vi "TA Main - Copy.vi"() -> ()   [LabVIEW 2019]
doc: "This example demonstrates how to acquire a continuous amount of data (Waveform) using the DAQ device's internal clock. It also shows how to synchronize two devices for different device families (E Series, S Series, M Series, X Series, DSA, and SC Express), to simultaneously acquire the data.\n\nFor instructions on how to connect your signals to the DAQ device, refer to your device documentation."
uses:
  Program Files/National Instruments/LabVIEW 2019/examples/Instrument IO/Serial/support/Serial - Settings.ctl
  <vilib>/Utility/error.llb/DialogType.ctl
  <vilib>/DAQmx/read.llb/DAQmx Read (Analog 1D Wfm NChan NSamp).vi
  <vilib>/Instr/_visa.llb/VISA Configure Serial Port (Instr).vi
  <vilib>/DAQmx/configure/timing.llb/DAQmx Timing (Sample Clock).vi
  <vilib>/DAQmx/configure/trigger.llb/DAQmx Start Trigger (Digital Edge).vi
  <vilib>/DAQmx/miscellaneous.llb/DAQmx Fill In Error Info.vi
panel:
  in  "Pass Logger":T1(tab)
  out "CO2 chart":waveform(dbl)[](graph)=[{"t0"=timestamp(3665042798.734879 s since 1904-01-01), "dt"=0.0, "Y"=[151.0], "attributes"=variant("NI_ChannelName"=variant(string "SCD30 CO2"), "NI_UnitDescription"=variant(string "ppm"))}, {"t0"=timestamp(3665042798.734879 s since 1904-01-01), "dt"=0.0, "Y"=[28.44], "attributes"=variant("NI_ChannelName"=variant(string "SCD30 Temp"), "NI_UnitDescription"=variant(string "C"))}, {"t0"=timestamp(3665042798.734879 s since 1904-01-01), "dt"=0.0, "Y"=[0.0], "attributes"=variant("NI_ChannelName"=variant(string "SCD30 Humidity"), "NI_UnitDescription"=variant(string "%"))}]
  in  "Stop":bool
  in  "Enable logging":bool caption="Enable"
  in  "File config":T2={"Filepath"=path "C:/Users/Administrator/Desktop/DAQ TA/Test data", "Test ID"="CO2_pulse_test_50sscm_1v5", "PC"="69DTQV2"}
  out "Lockin chart":waveform(dbl)[](graph)=[{"t0"=timestamp(3665042794.5437593 s since 1904-01-01), "dt"=4.999, "Y"=[-0.0029492353085881725], "attributes"=variant("NI_ChannelName"=variant(string "Phase - Mic Diff"), "NI_UnitDescription"=variant(string "Rad"))}, {"t0"=timestamp(3665042794.5437593 s since 1904-01-01), "dt"=4.999, "Y"=[2.2024304960006402], "attributes"=variant("NI_ChannelName"=variant(string "Amplitude - Mic Diff"), "NI_UnitDescription"=variant(string "Volts"))}]
  out "Lockin output 1":T3={"X"=1.1012104588247866, "Y"=-0.0032477381836216656, "R"=1.1012152480003201, "θ"=-0.0029492353085881725, "Amp"=2.2024304960006402, "dt"=4.999, "Active channel"="Mic Diff", "Ref channel"="Heater Voltage"} {"X" format="%#_3g"; "Y" format="%#_3g"; "R" format="%#_3g"}
  in  "Sampling config":cluster{"Fs":dbl, "#s":dbl}={"Fs"=1000.0, "#s"=5000.0} {"Fs" format="%.2p"}
  out "Readings":T4={"SCD30 CO2"=220.0, "SCD30 Temp (C)"=28.44, "SCD30 RH (%)"=0.0}
  out "Enable logging":bool
  in  "CO2 offset":dbl=69.0
  in  "Config 1":cluster{"Ref Index":i32, "Active Index":i32}={"Ref Index"=2, "Active Index"=5}
  out "Lockin output 5":T3={"X"=7.331709643282483, "Y"=0.49731099109465005, "R"=7.348556628023282, "θ"=0.06772641255423814, "Amp"=14.697113256046563, "dt"=4.999, "Active channel"="Heater Current", "Ref channel"="Heater Voltage"} {"X" format="%#_3g"; "Y" format="%#_3g"; "R" format="%#_3g"}
  out "Lockin output 6":T3={"X"=10.405708679082442, "Y"=0.4366095430141891, "R"=10.414864425761035, "θ"=0.04193405807955491, "Amp"=20.82972885152207, "dt"=4.999, "Active channel"="Heater Power", "Ref channel"="Heater Voltage"} {"X" format="%#_3g"; "Y" format="%#_3g"; "R" format="%#_3g"}
  out "Lockin output 4":T3={"X"=0.3532460188223979, "Y"=-0.0002886373096321914, "R"=0.35324613674514604, "θ"=-0.0008170997831991877, "Amp"=0.7064922734902921, "dt"=4.999, "Active channel"="Heater Voltage", "Ref channel"="Heater Voltage"} {"X" format="%#_3g"; "Y" format="%#_3g"; "R" format="%#_3g"}
  out "Lockin output 3":T3={"X"=1.1011542239382506, "Y"=-0.0034004178869849783, "R"=1.101159474253778, "θ"=-0.003088038899800522, "Amp"=2.202318948507556, "dt"=4.999, "Active channel"="Mic Active", "Ref channel"="Heater Voltage"} {"X" format="%#_3g"; "Y" format="%#_3g"; "R" format="%#_3g"}
  out "Lockin output 2":T3={"X"=-5.629936956115632e-05, "Y"=-0.00017491984854744577, "R"=0.00018375682961143246, "θ"=-1.8821838626707943, "Amp"=0.0003675136592228649, "dt"=4.999, "Active channel"="Mic Ref", "Ref channel"="Heater Voltage"} {"X" format="%#_3g"; "Y" format="%#_3g"; "R" format="%#_3g"}
  in  "Config 5":cluster{"Ref Index":i32, "Active Index":i32}={"Ref Index"=2, "Active Index"=6}
  in  "Config 4":cluster{"Ref Index":i32, "Active Index":i32}={"Ref Index"=2, "Active Index"=2}
  in  "Config 3":cluster{"Ref Index":i32, "Active Index":i32}={"Ref Index"=2, "Active Index"=1}
  in  "Config 2":cluster{"Ref Index":i32, "Active Index":i32}={"Ref Index"=2, "Active Index"=0}
  in  "Config 6":cluster{"Ref Index":i32, "Active Index":i32}={"Ref Index"=2, "Active Index"=8}
  out "Lockin output 1":T3={"X"=1.1012104588247866, "Y"=-0.0032477381836216656, "R"=1.1012152480003201, "θ"=-0.0029492353085881725, "Amp"=2.2024304960006402, "dt"=4.999, "Active channel"="Mic Diff", "Ref channel"="Heater Voltage"} {"X" format="%#_3g"; "Y" format="%#_3g"; "R" format="%#_3g"}
  in  "Config 7":cluster{"Ref Index":i32, "Active Index":i32}={"Ref Index"=2, "Active Index"=9}
  out "Lockin output 7":T3={"X"=5.973852436849716, "Y"=-22.75873151918968, "R"=23.529699813210815, "θ"=-1.3141009280278624, "Amp"=47.05939962642163, "dt"=4.999, "Active channel"="Heater Temp", "Ref channel"="Heater Voltage"} {"X" format="%#_3g"; "Y" format="%#_3g"; "R" format="%#_3g"}
  in  "Config 8":cluster{"Ref Index":i32, "Active Index":i32}={"Ref Index"=2, "Active Index"=7}
  out "Lockin output 8":T3={"X"=0.4029293718854757, "Y"=-1.4812546309068166, "R"=1.535078942696731, "θ"=-1.3052036543950893, "Amp"=3.070157885393462, "dt"=4.999, "Active channel"="Heater Resistance", "Ref channel"="Heater Voltage"} {"X" format="%#_3g"; "Y" format="%#_3g"; "R" format="%#_3g"}
  out "Lockin output 9":T3={"X"=-0.008023964066543083, "Y"=0.030564692860772787, "R"=0.03160038684912812, "θ"=1.8275270682644151, "Amp"=0.06320077369825625, "dt"=4.999, "Active channel"="Diode Voltage", "Ref channel"="Heater Voltage"} {"X" format="%#_3g"; "Y" format="%#_3g"; "R" format="%#_3g"}
  in  "Config 9":cluster{"Ref Index":i32, "Active Index":i32}={"Ref Index"=2, "Active Index"=4}
  in  "VISA resource name 2":refnum<visa-resource-name>="COM6"
  in  "Serial Settings":T5={"baud rate"=9600, "data bits"=8, "parity"=enum."None", "stop bits"=10, "flow control"=0} {"flow control" items=["None"=0, "XON/XOFF"=1, "RTS/CTS"=2, "DTR/DSR"=4]; "stop bits" items=["1.0"=10, "1.5"=15, "2.0"=20]; "data bits" min=5 max=8 step=1; "baud rate" items=["75"=75, "110"=110, "134"=134, "150"=150, "300"=300, "600"=600, "1200"=1200, "1800"=1800, "2400"=2400, "4800"=4800, "7200"=7200, "9600"=9600, "14400"=14400, "19200"=19200, "28800"=28800, "38400"=38400, "56000"=56000, "57600"=57600, "115200"=115200, "128000"=128000, "230400"=230400]}
  out "Waveform":waveform(dbl)(graph)={"t0"=timestamp(3665042794.5437374 s since 1904-01-01), "dt"=0.001, "Y"=array[5000 elements], "attributes"=variant("NI_ChannelName"=variant(string "Mic Diff"), "NI_UnitDescription"=variant(string "Volts"))}
  out "Channel names":T6={"Ref channel"="Mic Ref", "Active channel"="Mic Active"}
  in  "Config":T7={"Ref Index"=0, "Active Index"=1, "Gain"=1.0, "Channel name"="Mic Diff", "Enable"=TRUE, "Offset"=0.0035}
  in  "Filter config":T8={"Lower Cut-Off"=49.0, "Upper Cut-Off"=51.0}
  out "Noise estimate (mVrms)":dbl=53.14761345113184 format="%0.2f"
  out "Channel name":string="Diode Voltage"
  in  "Config":T9={"Channel Index"=4, "Diode TC (mV)"=-1.343, "Channel name"="Heater Temp", "Ref voltage"=0.8536, "Ref temp"=25.0} {"Ref temp" format="%.3f"; "Ref voltage" format="%.3f"; "Diode TC (mV)" format="%.3f"}
  out "AO Waveform Graph":waveform(dbl)(graph)={"t0"=timestamp(0 s since 1904-01-01), "dt"=0.001, "Y"=array[5000 elements]}
  in  "Channel config":T10={"Frequency"=47.0, "Voltage"=1.5, "Signal type"=enum."Sine Wave", "Square wave duty cycle (%)"=50.0, "physical channels"="Dev1/ao0", "name to assign"="Heater Voltage", "Phase"=-90.0} {"Square wave duty cycle (%)" format="%0.2f"}
  in  "Config":T11={"Voltage channel index"=2, "Shunt channel index"=3, "Shunt resistance"=10}
  out "Channel names":T12={"Voltage channel name"="Heater Voltage", "Shunt channel name"="Heater Shunt"}
  out "Diode Waveform":waveform(dbl)[](graph)=[{"t0"=timestamp(3665042794.5437374 s since 1904-01-01), "dt"=0.001, "Y"=array[5000 elements], "attributes"=variant("NI_ChannelName"=variant(string "Mic Ref"), "NI_UnitDescription"=variant(string "Volts"))}, {"t0"=timestamp(3665042794.5437484 s since 1904-01-01), "dt"=0.001, "Y"=array[5000 elements], "attributes"=variant("NI_ChannelName"=variant(string "Mic Active"), "NI_UnitDescription"=variant(string "Volts"))}, {"t0"=timestamp(3665042794.5437593 s since 1904-01-01), "dt"=0.001, "Y"=array[5000 elements], "attributes"=variant("NI_ChannelName"=variant(string "Heater Voltage"), "NI_UnitDescription"=variant(string "Volts"))}, {"t0"=timestamp(3665042794.5437703 s since 1904-01-01), "dt"=0.001, "Y"=array[5000 elements], "attributes"=variant("NI_ChannelName"=variant(string "Heater Shunt"), "NI_UnitDescription"=variant(string "Volts"))}, {"t0"=timestamp(3665042794.5437813 s since 1904-01-01), "dt"=0.001, "Y"=array[5000 elements], "attributes"=variant("NI_ChannelName"=variant(string "Diode Voltage"), "NI_UnitDescription"=variant(string "Volts"))}, {"t0"=timestamp(3665042794.5437374 s since 1904-01-01), "dt"=0.001, "Y"=array[5000 elements], "attributes"=variant("NI_ChannelName"=variant(string "Mic Diff"), "NI_UnitDescription"=variant(string "Volts"))}, {"t0"=timestamp(3665042794.5437703 s since 1904-01-01), "dt"=0.001, "Y"=array[5000 elements], "attributes"=variant("NI_ChannelName"=variant(string "Heater Current"), "NI_UnitDescription"=variant(string "mA"))}, {"t0"=timestamp(3665042794.5437593 s since 1904-01-01), "dt"=0.001, "Y"=array[5000 elements], "attributes"=variant("NI_ChannelName"=variant(string "Heater Resistance"), "NI_UnitDescription"=variant(string "Ohms"))}, {"t0"=timestamp(3665042794.5437593 s since 1904-01-01), "dt"=0.001, "Y"=array[5000 elements], "attributes"=variant("NI_ChannelName"=variant(string "Heater Power"), "NI_UnitDescription"=variant(string "mW"))}, {"t0"=timestamp(3665042794.5437813 s since 1904-01-01), "dt"=0.001, "Y"=array[5000 elements], "attributes"=variant("NI_ChannelName"=variant(string "Heater Temp"), "NI_UnitDescription"=variant(string "degC"))}]
  out "Microphone Waveform":waveform(dbl)[](graph)=[{"t0"=timestamp(3665042794.5437374 s since 1904-01-01), "dt"=0.001, "Y"=array[5000 elements], "attributes"=variant("NI_ChannelName"=variant(string "Mic Ref"), "NI_UnitDescription"=variant(string "Volts"))}, {"t0"=timestamp(3665042794.5437484 s since 1904-01-01), "dt"=0.001, "Y"=array[5000 elements], "attributes"=variant("NI_ChannelName"=variant(string "Mic Active"), "NI_UnitDescription"=variant(string "Volts"))}, {"t0"=timestamp(3665042794.5437593 s since 1904-01-01), "dt"=0.001, "Y"=array[5000 elements], "attributes"=variant("NI_ChannelName"=variant(string "Heater Voltage"), "NI_UnitDescription"=variant(string "Volts"))}, {"t0"=timestamp(3665042794.5437703 s since 1904-01-01), "dt"=0.001, "Y"=array[5000 elements], "attributes"=variant("NI_ChannelName"=variant(string "Heater Shunt"), "NI_UnitDescription"=variant(string "Volts"))}, {"t0"=timestamp(3665042794.5437813 s since 1904-01-01), "dt"=0.001, "Y"=array[5000 elements], "attributes"=variant("NI_ChannelName"=variant(string "Diode Voltage"), "NI_UnitDescription"=variant(string "Volts"))}, {"t0"=timestamp(3665042794.5437374 s since 1904-01-01), "dt"=0.001, "Y"=array[5000 elements], "attributes"=variant("NI_ChannelName"=variant(string "Mic Diff"), "NI_UnitDescription"=variant(string "Volts"))}, {"t0"=timestamp(3665042794.5437703 s since 1904-01-01), "dt"=0.001, "Y"=array[5000 elements], "attributes"=variant("NI_ChannelName"=variant(string "Heater Current"), "NI_UnitDescription"=variant(string "mA"))}, {"t0"=timestamp(3665042794.5437593 s since 1904-01-01), "dt"=0.001, "Y"=array[5000 elements], "attributes"=variant("NI_ChannelName"=variant(string "Heater Resistance"), "NI_UnitDescription"=variant(string "Ohms"))}, {"t0"=timestamp(3665042794.5437593 s since 1904-01-01), "dt"=0.001, "Y"=array[5000 elements], "attributes"=variant("NI_ChannelName"=variant(string "Heater Power"), "NI_UnitDescription"=variant(string "mW"))}, {"t0"=timestamp(3665042794.5437813 s since 1904-01-01), "dt"=0.001, "Y"=array[5000 elements], "attributes"=variant("NI_ChannelName"=variant(string "Heater Temp"), "NI_UnitDescription"=variant(string "degC"))}]
  out "Heater Waveform":waveform(dbl)[](graph)=[{"t0"=timestamp(3665042794.5437374 s since 1904-01-01), "dt"=0.001, "Y"=array[5000 elements], "attributes"=variant("NI_ChannelName"=variant(string "Mic Ref"), "NI_UnitDescription"=variant(string "Volts"))}, {"t0"=timestamp(3665042794.5437484 s since 1904-01-01), "dt"=0.001, "Y"=array[5000 elements], "attributes"=variant("NI_ChannelName"=variant(string "Mic Active"), "NI_UnitDescription"=variant(string "Volts"))}, {"t0"=timestamp(3665042794.5437593 s since 1904-01-01), "dt"=0.001, "Y"=array[5000 elements], "attributes"=variant("NI_ChannelName"=variant(string "Heater Voltage"), "NI_UnitDescription"=variant(string "Volts"))}, {"t0"=timestamp(3665042794.5437703 s since 1904-01-01), "dt"=0.001, "Y"=array[5000 elements], "attributes"=variant("NI_ChannelName"=variant(string "Heater Shunt"), "NI_UnitDescription"=variant(string "Volts"))}, {"t0"=timestamp(3665042794.5437813 s since 1904-01-01), "dt"=0.001, "Y"=array[5000 elements], "attributes"=variant("NI_ChannelName"=variant(string "Diode Voltage"), "NI_UnitDescription"=variant(string "Volts"))}, {"t0"=timestamp(3665042794.5437374 s since 1904-01-01), "dt"=0.001, "Y"=array[5000 elements], "attributes"=variant("NI_ChannelName"=variant(string "Mic Diff"), "NI_UnitDescription"=variant(string "Volts"))}, {"t0"=timestamp(3665042794.5437703 s since 1904-01-01), "dt"=0.001, "Y"=array[5000 elements], "attributes"=variant("NI_ChannelName"=variant(string "Heater Current"), "NI_UnitDescription"=variant(string "mA"))}, {"t0"=timestamp(3665042794.5437593 s since 1904-01-01), "dt"=0.001, "Y"=array[5000 elements], "attributes"=variant("NI_ChannelName"=variant(string "Heater Resistance"), "NI_UnitDescription"=variant(string "Ohms"))}, {"t0"=timestamp(3665042794.5437593 s since 1904-01-01), "dt"=0.001, "Y"=array[5000 elements], "attributes"=variant("NI_ChannelName"=variant(string "Heater Power"), "NI_UnitDescription"=variant(string "mW"))}, {"t0"=timestamp(3665042794.5437813 s since 1904-01-01), "dt"=0.001, "Y"=array[5000 elements], "attributes"=variant("NI_ChannelName"=variant(string "Heater Temp"), "NI_UnitDescription"=variant(string "degC"))}]
  in  "Channel 4 config":T13={"Channel"="Dev1/ai3", "Vmax"=0.5, "Vmin"=0.0, "name to assign"="Heater Shunt", "input terminal configuration"=10106} {"input terminal configuration" items=["Default"=-1, "RSE"=10083, "NRSE"=10078, "Differential"=10106, "Pseudodifferential"=12529]; "Vmin" format="%0.2f"; "Vmax" format="%0.2f"}
  in  "Channel 3 config":T13={"Channel"="Dev1/ai2", "Vmax"=3.0, "Vmin"=0.0, "name to assign"="Heater Voltage", "input terminal configuration"=10106} {"input terminal configuration" items=["Default"=-1, "RSE"=10083, "NRSE"=10078, "Differential"=10106, "Pseudodifferential"=12529]; "Vmin" format="%0.2f"; "Vmax" format="%0.2f"}
  in  "Channel 2 config":T13={"Channel"="Dev1/ai1", "Vmax"=3.0, "Vmin"=-3.0, "name to assign"="Mic Active", "input terminal configuration"=10083} {"input terminal configuration" items=["Default"=-1, "RSE"=10083, "NRSE"=10078, "Differential"=10106, "Pseudodifferential"=12529]; "Vmin" format="%0.2f"; "Vmax" format="%0.2f"}
  in  "Channel 1 config":T13={"Channel"="Dev1/ai0", "Vmax"=3.0, "Vmin"=-3.0, "name to assign"="Mic Ref", "input terminal configuration"=10083} {"input terminal configuration" items=["Default"=-1, "RSE"=10083, "NRSE"=10078, "Differential"=10106, "Pseudodifferential"=12529]; "Vmin" format="%0.2f"; "Vmax" format="%0.2f"}
  in  "Channel 5 config":T13={"Channel"="Dev1/ai4", "Vmax"=1.0, "Vmin"=0.0, "name to assign"="Diode Voltage", "input terminal configuration"=10083} {"input terminal configuration" items=["Default"=-1, "RSE"=10083, "NRSE"=10078, "Differential"=10106, "Pseudodifferential"=12529]; "Vmin" format="%0.2f"; "Vmax" format="%0.2f"}
  # "PAS Logger"
  # "(ppm)"
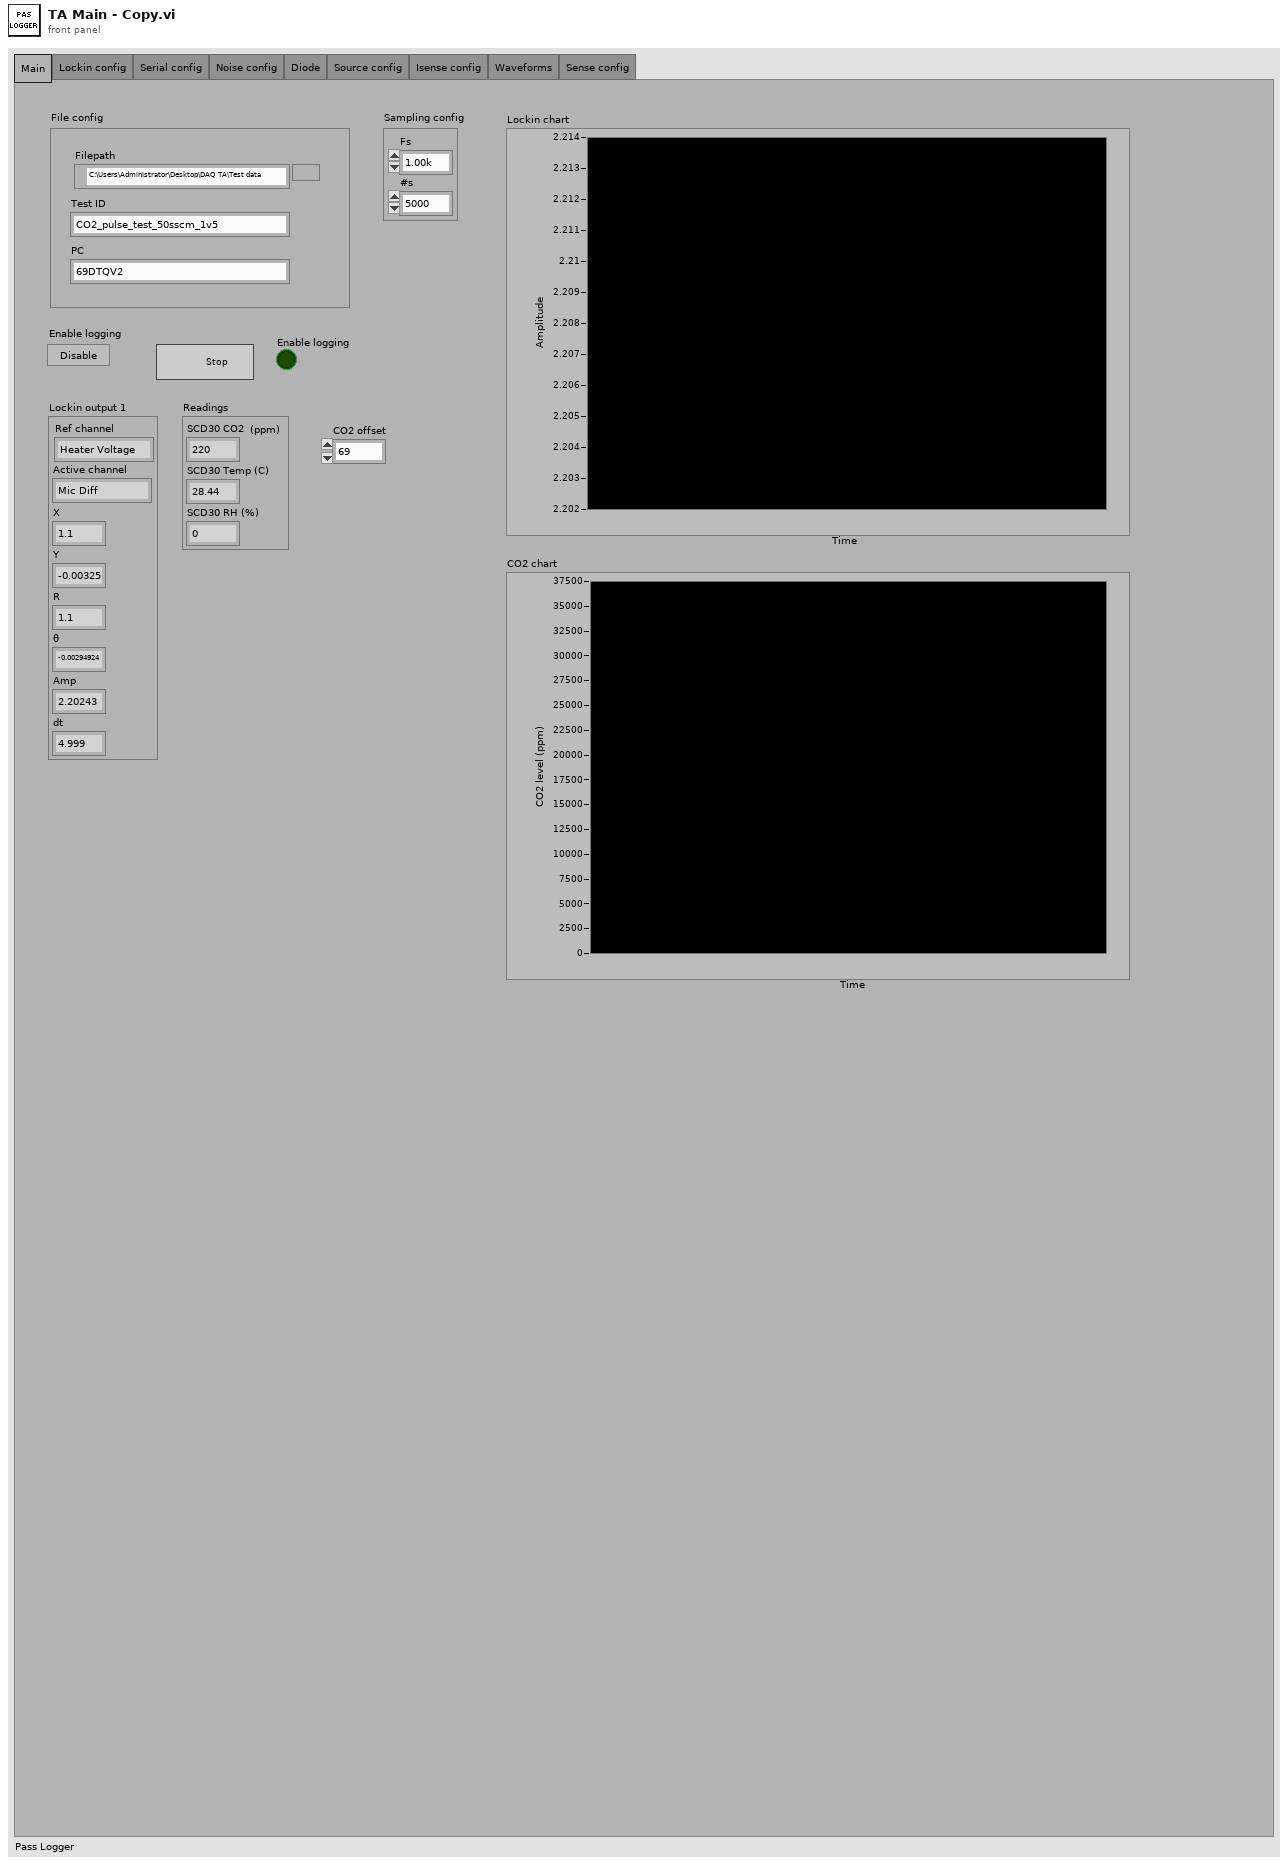
[diagram p1: front panel]
types:
  T1 = enum32{"Main", "Lockin config", "Serial config", "Noise config", "Diode", "Source config", "Isense config", "Waveforms", "Sense config"}
  T2 = cluster{"Filepath":path, "Test ID":string, "PC":string}
  T3 = cluster{"X":dbl, "Y":dbl, "R":dbl, "θ":dbl, "Amp":dbl, "dt":dbl, "Active channel":string, "Ref channel":string}
  T4 = cluster{"SCD30 CO2":dbl, "SCD30 Temp (C)":dbl, "SCD30 RH (%)":dbl}
  T5 = typedef "Serial - Settings.ctl" = cluster{"baud rate":u32, "data bits":u16, "parity":enum16{"None", "Odd", "Even", "Mark", "Space"}, "stop bits":u16, "flow control":u16}
  T6 = cluster{"Ref channel":string, "Active channel":string}
  T7 = cluster{"Ref Index":i32, "Active Index":i32, "Gain":dbl, "Channel name":string, "Enable":bool, "Offset":dbl}
  T8 = cluster{"Lower Cut-Off":dbl, "Upper Cut-Off":dbl}
  T9 = cluster{"Channel Index":i32, "Diode TC (mV)":dbl, "Channel name":string, "Ref voltage":dbl, "Ref temp":dbl}
  T10 = cluster{"Frequency":dbl, "Voltage":dbl, "Signal type":enum16{"Sine Wave", "Triangle Wave", "Square Wave", "Sawtooth Wave"}, "Square wave duty cycle (%)":dbl, "physical channels":tag, "name to assign":string, "Phase":dbl}
  T11 = cluster{"Voltage channel index":i32, "Shunt channel index":i32, "Shunt resistance":i32}
  T12 = cluster{"Voltage channel name":string, "Shunt channel name":string}
  T13 = cluster{"Channel":tag, "Vmax":dbl, "Vmin":dbl, "name to assign":string, "input terminal configuration":i32}
  T14 = cluster{"Active channel":string, "Ref channel":string}
  T15 = typedef "DialogType.ctl" = u16
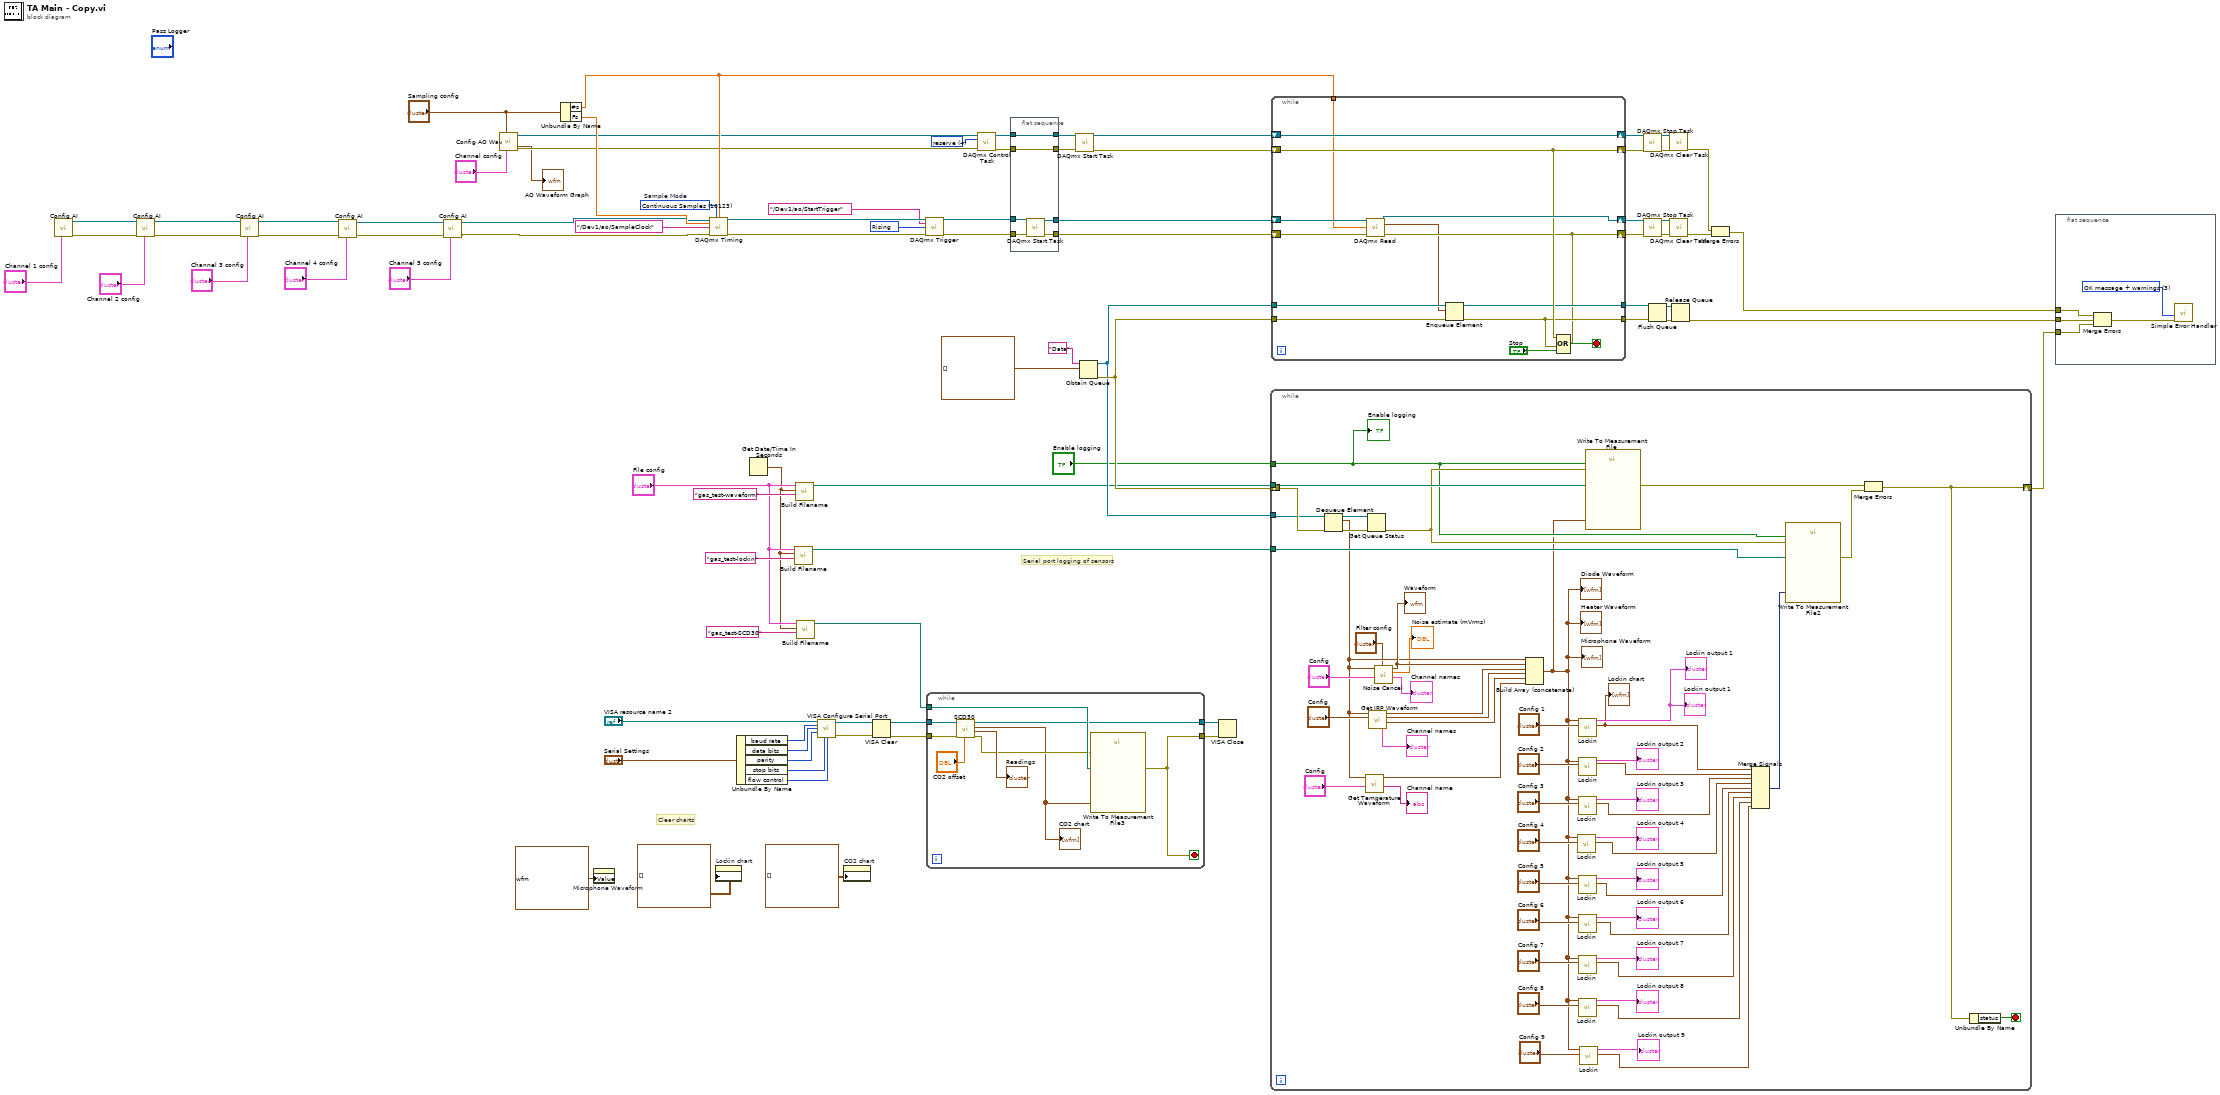
[diagram p0: block diagram]
diagram:
  w67 = 10280 items=["Rising"=10280, "Falling"=10171] ("edge")
  w74 = 4 items=["verify"=2, "reserve"=4, "commit"=3, "unreserve"=5, "abort"=6] ("action")
  w75 = 10123 items=["Finite Samples"=10178, "Continuous Samples"=10123, "Hardware Timed Single Point"=12522]  # Sample Mode
  # "Clear charts"
  # "Serial port logging of sensors"
  n1 = call "Config AI.vi"("Channel config"="Channel 1 config") -> ("error out"=w58:errorcluster, "task out"=w57:refnum<k21>)  [unwired: 9 in]
  n2 = call "Config AI.vi"("Channel config"="Channel 2 config", "error in"=w58, "task in"=w57) -> ("error out"=w12:errorcluster, "task out"=w11:refnum<k21>)  [unwired: 7 in]
  n3 = call "Config AI.vi"("Channel config"="Channel 3 config", "error in"=w12, "task in"=w11) -> ("error out"=w43:errorcluster, "task out"=w42:refnum<k21>)  [unwired: 7 in]
  n4 = call "Config AI.vi"("Channel config"="Channel 4 config", "error in"=w43, "task in"=w42) -> ("error out"=w5:errorcluster, "task out"=w4:refnum<k21>)  [unwired: 7 in]
  n5 = call "Config AI.vi"("Channel config"="Channel 5 config", "error in"=w5, "task in"=w4) -> ("error out"=w2:errorcluster, "task out"=w3:refnum<k21>)  [unwired: 7 in]
  n6 = call "Config AO Wav.vi"("Channel config"="Channel config", "Sampling info"="Sampling config") -> ("error out"=w9:errorcluster, "task out"=w10:refnum<k21>, "AO Waveform Graph"=→"AO Waveform Graph":waveform(dbl))  [unwired: 7 in]
  n7 = Unbundle By Name("Sampling config") -> ("#s"=w45:dbl, "Fs"=w44:dbl)
  n8 = property on="Microphone Waveform" class="WFGraph (strict)"("Value"=waveform(dbl)[] [{"t0"=timestamp(3651561790.263236 s since 1904-01-01), "dt"=0.001, "Y"=array[2000 elements], "attributes"=variant("NI_ChannelName"=variant(string "Mic Active"), "NI_UnitDescription"=variant(string "Volts"))}, {"t0"=timestamp(3651561790.263247 s since 1904-01-01), "dt"=0.001, "Y"=array[2000 elements], "attributes"=variant("NI_ChannelName"=variant(string "Mic Ref"), "NI_UnitDescription"=variant(string "Volts"))}, {"t0"=timestamp(3651561790.263258 s since 1904-01-01), "dt"=0.001, "Y"=array[2000 elements], "attributes"=variant("NI_ChannelName"=variant(string "Diode Heater"), "NI_UnitDescription"=variant(string "Volts"))}, {"t0"=timestamp(3651561790.263269 s since 1904-01-01), "dt"=0.001, "Y"=array[2000 elements], "attributes"=variant("NI_ChannelName"=variant(string "Diode Amb"), "NI_UnitDescription"=variant(string "Volts"))}, {"t0"=timestamp(3651561790.26328 s since 1904-01-01), "dt"=0.001, "Y"=array[2000 elements], "attributes"=variant("NI_ChannelName"=variant(string "Heater Shunt"), "NI_UnitDescription"=variant(string "Volts"))}, {"t0"=timestamp(3651561790.2632914 s since 1904-01-01), "dt"=0.001, "Y"=array[2000 elements], "attributes"=variant("NI_ChannelName"=variant(string "Heater V"), "NI_UnitDescription"=variant(string "Volts"))}, {"t0"=timestamp(3651561790.263247 s since 1904-01-01), "dt"=0.001, "Y"=array[2000 elements], "attributes"=variant("NI_ChannelName"=variant(string "Mic Diff"), "NI_UnitDescription"=variant(string "Volts"))}, {"t0"=timestamp(3651561790.26328 s since 1904-01-01), "dt"=0.001, "Y"=array[2000 elements], "attributes"=variant("NI_ChannelName"=variant(string "Heater Current"), "NI_UnitDescription"=variant(string "Amps"))}] ("Waveform")) -> ()  [unwired: 2 in, 2 out]
  n9 = call-poly <vilib>:"DAQmx Timing.vi"("task/channels in"=w3, "sample mode"=w75, "samples per channel"=w45, "rate"=w44, "source"=tag "/Dev1/ao/SampleClock", "error in"=w2) -> ("task out"=w68:refnum<k21>, "error out"=w69:errorcluster)  [unwired: 8 in]
  n10 = property on="Lockin chart" class="WFChart (strict)"("History Data"=waveform(dbl)[][] []) -> ()  [unwired: 2 in, 2 out]
  n11 = Unbundle By Name("Serial Settings") -> ("baud rate"=w27:u32, "data bits"=w26:u16, "parity"=w25:enum16{"None", "Odd", "Even", "Mark", "Space"}, "stop bits"=w24:u16, "flow control"=w23:u16)
  n12 = Get Date/Time In Seconds() -> (seconds since 1Jan1904=w30:timestamp)
  n13 = call "Build Filename.vi"("Test type"="gas_test-lockin" ("File Descriptor"), "time stamp"=w30, "File config"="File config") -> ("appended path"=w33:path)  [unwired: 8 in]
  n14 = call "Build Filename.vi"("Test type"="gas_test-waveform" ("File type"), "time stamp"=w30, "File config"="File config") -> ("appended path"=w35:path)  [unwired: 8 in]
  n15 = call "Build Filename.vi"("Test type"="gas_test-SCD30" ("File Descriptor"), "time stamp"=w30, "File config"="File config") -> ("appended path"=w16:path)  [unwired: 8 in]
  n16 = call-poly "VISA Configure Serial Port"("VISA resource name"="VISA resource name 2", "baud rate (9600)"=w27, "data bits (8)"=w26, "parity (0:none)"=w25, "stop bits (10: 1 bit)"=w24, "flow control (0:none)"=w23) -> ("VISA resource name out"=w21:refnum<visa-resource-name>, "error out"=w22:errorcluster)  [unwired: 3 in, 5 out]
  n17 = property on="CO2 chart" class="WFChart (strict)"("History Data"=waveform(dbl)[][] []) -> ()  [unwired: 2 in, 2 out]
  n18 = VISA Clear(VISA resource name=w21, error in (no error)=w22) -> (VISA resource name out=w20:refnum<visa-resource-name>, error out=w19:errorcluster)
  n19 = call-poly <vilib>:"DAQmx Trigger.vi"("task/channels in"=w68, "source"=tag "/Dev1/ao/StartTrigger", "edge"=w67, "error in"=w69) -> ("task out"=w65:refnum<k21>, "error out"=w66:errorcluster)  [unwired: 10 in]
  n20 = while {
    tunnel: w20 -> [w92]
    tunnel: w19 -> [w91]
    tunnel: [w93] -> w18
    tunnel: [w87] -> w17
    tunnel: w16 -> [w94]
    stop <- w93 stop-if-true
    n21 = call "SCD30.vi"("CO2 offset"="CO2 offset", "error in (no error)"=w91, "VISA resource name"=w92) -> ("error out"=w89:errorcluster, "Readings"=→"Readings":T4, "appended array"=w88:waveform(dbl)[], "VISA resource name out"=w87:refnum<visa-resource-name>)  [unwired: 5 in]
    "CO2 chart" <- w88
    n22 = call "Write To Measurement File3"("Signals"=w88, "error in (no error)"=w89, "Filename"=w94) -> ("error out"=w93:errorcluster)  [unwired: 14 in, 2 out]
  }
  n23 = call <vilib>:"DAQmx Control Task.vi"("task/channels in"=w10, "action"=w74, "error in"=w9) -> ("task out"=w64:refnum<k21>, "error out"=w62:errorcluster)  [unwired: 11 in]
  n24 = flat-sequence {
    tunnel: [w100] -> w71
    tunnel: [w99] -> w70
    tunnel: w66 -> [w98]
    tunnel: w65 -> [w97]
    tunnel: w64 -> [w96]
    tunnel: [w96] -> w63
    tunnel: w62 -> [w95]
    tunnel: [w95] -> w61
    frame #0 {
      n25 = call <vilib>:"DAQmx Start Task.vi"("task/channels in"=w97, "error in"=w98) -> ("task out"=w99:refnum<k21>, "error out"=w100:errorcluster)  [unwired: 12 in]
    }
  }
  n26 = call <vilib>:"DAQmx Start Task.vi"("task/channels in"=w63, "error in"=w61) -> ("task out"=w72:refnum<k21>, "error out"=w73:errorcluster)  [unwired: 12 in]
  n27 = Obtain Queue(name (unnamed)="Data" ("名前（名前なし）"), element data type=waveform(dbl)[] [] ("data")) -> (queue out=w48:refnum<queue>, error out=w49:errorcluster)  [unwired: 3 in, 1 out]
  n28 = VISA Close(VISA resource name=w17, error in (no error)=w18) -> ()  [unwired: 1 out]
  n29 = while {
    tunnel: w48 -> [w154]
    shift-right: [w145] -> w47
    shift-left: w49 -> [w155]
    tunnel: w35 -> [w153]
    tunnel: "Enable logging" -> [w149]
    tunnel: w33 -> [w148]
    stop <- w141 stop-if-true
    n30 = Dequeue Element(queue=w154, error in (no error)=w155) -> (queue out=w151:refnum<queue>, element=w110:waveform(dbl)[], error out=w152:errorcluster)  [unwired: 1 in, 1 out]
    n31 = call "Get Temperature Waveform.vi"("Config"="Config", "array"=w110) -> ("Channel name"=→"Channel name":string, "waveform out"=w109:waveform(dbl))  [unwired: 8 in]
    n32 = Get Queue Status(queue=w151, error in (no error)=w152) -> (error out=w150:errorcluster)  [unwired: 1 in, 7 out]
    n33 = call "Get IRP Waveform.vi"("Channel config"="Config", "array"=w110) -> ("Power waveform out"=w119:waveform(dbl), "Resistance waveform out"=w120:waveform(dbl), "Current waveform out"=w122:waveform(dbl), "Channel names"=→"Channel names":T12)  [unwired: 6 in]
    n34 = call "Noise Cancel.vi"("Filter config"="Filter config", "Config"="Config", "array"=w110) -> ("Channel names"=→"Channel names":T14, "Noise estimate (mVrms)"=→"Noise estimate (mVrms)":dbl, "waveform out"=w143:waveform(dbl))  [unwired: 6 in]
    "Waveform" <- w143
    n35 = Build Array (concatenate)(w110, w143, w122, w120, w119, w109) -> (w103:waveform(dbl)[])
    "Microphone Waveform" <- w103
    "Heater Waveform" <- w103
    "Diode Waveform" <- w103
    n36 = call "Lockin.vi"("Config"="Config 4", "array"=w103) -> ("Output waveform"=w137:waveform(dbl)[], "Lockin output"=→"Lockin output 4":T3)  [unwired: 8 in]
    n37 = call "Lockin.vi"("Config"="Config 3", "array"=w103) -> ("Output waveform"=w138:waveform(dbl)[], "Lockin output"=→"Lockin output 3":T3)  [unwired: 8 in]
    n38 = call "Lockin.vi"("Config"="Config 5", "array"=w103) -> ("Output waveform"=w136:waveform(dbl)[], "Lockin output"=→"Lockin output 5":T3)  [unwired: 8 in]
    n39 = call "Lockin.vi"("Config"="Config 6", "array"=w103) -> ("Output waveform"=w135:waveform(dbl)[], "Lockin output"=→"Lockin output 6":T3)  [unwired: 8 in]
    n40 = call "Lockin.vi"("Config"="Config 7", "array"=w103) -> ("Output waveform"=w115:waveform(dbl)[], "Lockin output"=→"Lockin output 7":T3)  [unwired: 8 in]
    n41 = call "Lockin.vi"("Config"="Config 8", "array"=w103) -> ("Output waveform"=w111:waveform(dbl)[], "Lockin output"=→"Lockin output 8":T3)  [unwired: 8 in]
    n42 = call "Lockin.vi"("Config"="Config 1", "array"=w103) -> ("Output waveform"=w106:waveform(dbl)[], "Lockin output"=→"Lockin output 1" →"Lockin output 1":T3)  [unwired: 8 in]
    "Lockin chart" <- w106
    n43 = call "Lockin.vi"("Config"="Config 2", "array"=w103) -> ("Output waveform"=w139:waveform(dbl)[], "Lockin output"=→"Lockin output 2":T3)  [unwired: 8 in]
    n44 = call "Lockin.vi"("Config"="Config 9", "array"=w103) -> ("Output waveform"=w102:waveform(dbl)[], "Lockin output"=→"Lockin output 9":T3)  [unwired: 8 in]
    n45 = call "Write To Measurement File"("Signals"=w103, "Enable"=w149, "error in (no error)"=w150, "Filename"=w153) -> ("error out"=w146:errorcluster)  [unwired: 13 in, 2 out]
    n46 = Merge Signals(w106, w139, w138, w137, w136, w135, w115, w111, w102) -> (w134:dynamicdata)
    n47 = call "Write To Measurement File2"("Signals"=w134, "Enable"=w149, "error in (no error)"=w150, "Filename"=w148) -> ("error out"=w147:errorcluster)  [unwired: 13 in, 2 out]
    n48 = Merge Errors(w146, w147) -> (w145:errorcluster)
    n49 = Unbundle By Name(w145) -> ("status"=w141:bool)
    "Enable logging" <- w149
  }
  n50 = while {
    shift-right: [w165] -> w84
    shift-left: w73 -> [w165]
    shift-right: [w157] -> w80
    shift-left: w71 -> [w167]
    shift-right: [w164] -> w85
    shift-left: w72 -> [w164]
    shift-right: [w166] -> w81
    shift-left: w70 -> [w168]
    tunnel: w45 -> [w163]
    tunnel: [w162] -> w54
    tunnel: [w158] -> w53
    tunnel: w48 -> [w161]
    tunnel: w49 -> [w160]
    stop <- w169 stop-if-true
    n51 = call-poly <vilib>:"DAQmx Read.vi"("task/channels in"=w168, "number of samples per channel"=w163, "error in"=w167) -> ("task out"=w166:refnum<k21>, "data"=w156:waveform(dbl)[], "error out"=w157:errorcluster)  [unwired: 10 in]
    n52 = Enqueue Element(queue=w161, element=w156, error in (no error)=w160) -> (queue out=w162:refnum<queue>, error out=w158:errorcluster)  [unwired: 1 in, 1 out]
    n53 = Compound Arithmetic op=OR(w165, w157, w158, "Stop") -> (w169:bool)
  }
  n54 = call <vilib>:"DAQmx Stop Task.vi"("task/channels in"=w85, "error in"=w84) -> ("task out"=w82:refnum<k21>, "error out"=w83:errorcluster)  [unwired: 12 in]
  n55 = call <vilib>:"DAQmx Stop Task.vi"("task/channels in"=w81, "error in"=w80) -> ("task out"=w78:refnum<k21>, "error out"=w79:errorcluster)  [unwired: 12 in]
  n56 = Flush Queue(queue=w54, error in (no error)=w53) -> (queue out=w55:refnum<queue>, error out=w56:errorcluster)  [unwired: 1 out]
  n57 = call <vilib>:"DAQmx Clear Task.vi"("task in"=w82, "error in"=w83) -> ("error out"=w77:errorcluster)  [unwired: 13 in]
  n58 = call <vilib>:"DAQmx Clear Task.vi"("task in"=w78, "error in"=w79) -> ("error out"=w76:errorcluster)  [unwired: 13 in]
  n59 = Release Queue(queue=w55, error in (no error)=w56) -> (error out=w51:errorcluster)  [unwired: 1 in, 2 out]
  n60 = Merge Errors(w77, w76) -> (w52:errorcluster)
  n61 = flat-sequence {
    tunnel: w52 -> [w174]
    tunnel: w51 -> [w173]
    tunnel: w47 -> [w170]
    frame #0 {
      w172 = T15 3 items=["no dialog", "OK message", "continue or stop message", "OK message + warnings", "continue/stop + warnings"] ("type of dialog (OK msg:1)")
      n62 = Merge Errors(w174, w173, w170) -> (w171:errorcluster)
      n63 = call <vilib>:"Simple Error Handler.vi"("type of dialog (OK msg:1)"=w172, "error in (no error)"=w171) -> ()  [unwired: 3 in, 5 out]
    }
  }
